vi "Set Finger Forces.vi"(8 "error in (no error)":errorcluster, 10 "Finger Forces":T1, 11 "MF3 in":refnum<class "MF3.lvclass">) -> (0 "error out":errorcluster, 2 "Current setpoints":dbl[](array[numeric]) format="%.2f", 3 "MF3 out":refnum<class "MF3.lvclass">)   [LabVIEW 2011, in "MF3.lvclass"]
uses:
  MF3.lvclass
  Controls/Motor Names.ctl
  MF3.lvclass/MF3.ctl
  <vilib>/Analysis/Matrix/Numeric/Multiply/Multiply - RM,RM.vi
  Finger/Finger.lvclass
  <vilib>/Analysis/Matrix/NI_Matrix.lvlib
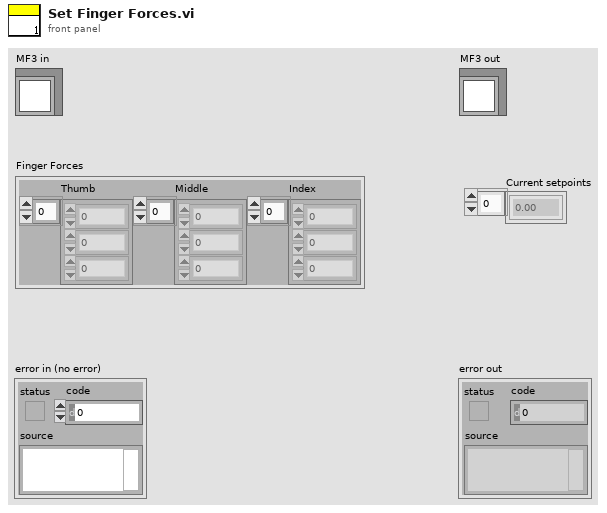
[diagram p1: front panel]
types:
  T1 = cluster{"Thumb":dbl[], "Middle":dbl[], "Index":dbl[]}
  T2 = typedef "Motor Names.ctl" = enum16{"Thumb1", "Thumb2", "Thumb3", "Middle1", "Middle2", "Middle3", "Redundant", "Index1", "Index2", "Index3"}
  T3 = typedef "NI_Matrix.lvlib/RealMatrix.ctl" = dbl[][]
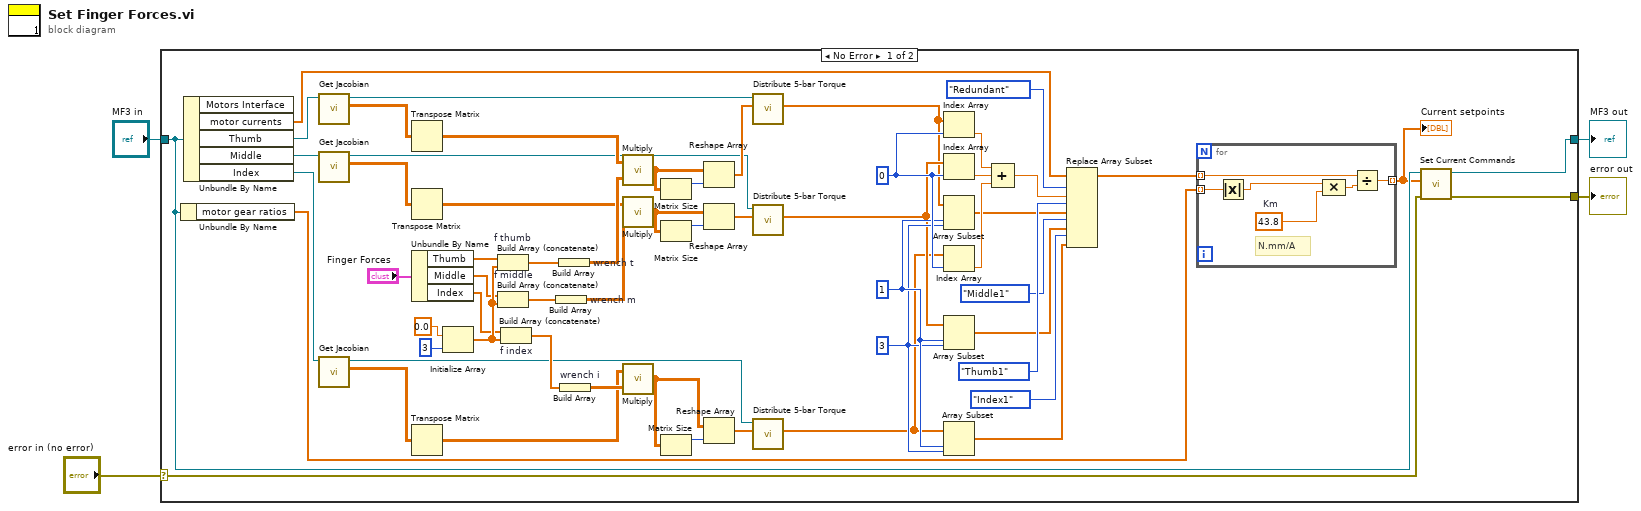
[diagram p0: block diagram]
diagram:
  n1 = case shown="No Error" "error in (no error)" {
    selector: "error in (no error)" -> [w8 w71]
    tunnel: [w7 w71] -> w3
    tunnel: [w6 w70] -> w1
    tunnel: "MF3 in" -> [w9 w70]
    frame No Error {
      w26 = 3 ("length")
      w27 = 1 ("index")
      w31 = 0 ("index")
      n2 = Unbundle By Name(w9) -> ("motor gear ratios"=w14:dbl[])
      n3 = Unbundle By Name(w9) -> ("motor currents"=w19:dbl[], "Thumb"=w63:refnum<class "Finger.lvclass">, "Middle"=w62:refnum<class "Finger.lvclass">, "Index"=w61:refnum<class "Finger.lvclass">)  [unwired: 1 out]
      n4 = call "Get Jacobian.vi"("Finger in"=w63) -> ("Jacobian"=w51:T3, "Finger out"=w35:refnum<class "Finger.lvclass">)  [unwired: 8 in, 1 out]
      n5 = call "Get Jacobian.vi"("Finger in"=w62) -> ("Jacobian"=w52:T3, "Finger out"=w34:refnum<class "Finger.lvclass">)  [unwired: 8 in, 1 out]
      n6 = call "Get Jacobian.vi"("Finger in"=w61) -> ("Jacobian"=w53:T3, "Finger out"=w33:refnum<class "Finger.lvclass">)  [unwired: 8 in, 1 out]
      n7 = Transpose Matrix(1:w51) -> (0:w50:T3)
      n8 = Transpose Matrix(1:w52) -> (0:w48:T3)
      n9 = Unbundle By Name("Finger Forces") -> ("Thumb"=w10:dbl[], "Middle"=w11:dbl[], "Index"=w12:dbl[])
      n10 = Transpose Matrix(1:w53) -> (0:w45:T3)
      n11 = Initialize Array(0.0 ("element"), 3 ("dimension size")) -> (w57:dbl[])
      n12 = Build Array (concatenate) "f thumb"(w10, w57) -> (w56:dbl[])
      n13 = Build Array (concatenate) "f middle"(w11, w57) -> (w55:dbl[])
      n14 = Build Array (concatenate) "f index"(w12, w57) -> (w54:dbl[])
      n15 = Build Array "wrench m"(w55) -> (w47:T3)
      n16 = Build Array "wrench t"(w56) -> (w49:T3)
      n17 = Build Array "wrench i"(w54) -> (w46:T3)
      n18 = call-poly <vilib>:"Multiply.vi"("Real Matrix B"=w49, "Real Matrix A"=w50) -> ("A * B"=w43:T3)
      n19 = call-poly <vilib>:"Multiply.vi"("Real Matrix B"=w47, "Real Matrix A"=w48) -> ("A * B"=w41:T3)
      n20 = call-poly <vilib>:"Multiply.vi"("Real Matrix B"=w46, "Real Matrix A"=w45) -> ("A * B"=w39:T3)
      n21 = Matrix Size(0:w43) -> (1:w44:i32)  [unwired: 1 out]
      n22 = Matrix Size(0:w41) -> (1:w42:i32)  [unwired: 1 out]
      n23 = Matrix Size(0:w39) -> (1:w40:i32)  [unwired: 1 out]
      n24 = Reshape Array(w43, w44) -> (w36:dbl[])
      n25 = Reshape Array(w41, w42) -> (w37:dbl[])
      n26 = Reshape Array(w39, w40) -> (w38:dbl[])
      n27 = call "Distribute 5-bar Torque.vi"("joint_torques"=w36, "Finger in"=w35) -> ("motor_torques"=w23:dbl[])  [unwired: 7 in, 2 out]
      n28 = call "Distribute 5-bar Torque.vi"("joint_torques"=w37, "Finger in"=w34) -> ("motor_torques"=w25:dbl[])  [unwired: 7 in, 2 out]
      n29 = call "Distribute 5-bar Torque.vi"("joint_torques"=w38, "Finger in"=w33) -> ("motor_torques"=w24:dbl[])  [unwired: 7 in, 2 out]
      n30 = Index Array(array=w23, index=w31) -> (element=w32:dbl)
      n31 = Index Array(array=w25, index=w31) -> (element=w29:dbl)
      n32 = Array Subset(array=w23, index=w27, length=w26) -> (w17:dbl[])
      n33 = Index Array(array=w24, index=w31) -> (element=w30:dbl)
      n34 = Array Subset(array=w25, index=w27, length=w26) -> (w16:dbl[])
      n35 = Array Subset(array=w24, index=w27, length=w26) -> (w15:dbl[])
      n36 = Compound Arithmetic op=ADD(w32, w29, w30) -> (w18:dbl)
      n37 = Replace Array Subset "Replace Array Subset"(array=w19, new element #1=w18, index #1=Motor_Names."Redundant" ("Motor Names"), new element #2=w17, index #2=Motor_Names."Thumb1" ("Motor Names"), new element #3=w16, index #3=Motor_Names."Middle1" ("Motor Names"), new element #4=w15, index #4=Motor_Names."Index1" ("Motor Names")) -> (w13:dbl[])
      n38 = for {
        tunnel: w14 -> [w65] mode=indexing
        tunnel: w13 -> [w69] mode=indexing
        tunnel: [w67] -> w5 mode=indexing
        w64 = 43.8  # Km
        # "N.mm/A"
        n39 = Absolute Value(x=w65) -> (abs(x)=w66:dbl)
        n40 = Compound Arithmetic op=MULTIPLY(w66, w64) -> (w68:dbl)
        n41 = Divide(x=w69, y=w68) -> (x/y=w67:dbl)
      }
      "Current setpoints" <- w5
      n42 = call "Set Current Commands.vi"("error in (no error)"=w8, "current commands"=w5, "MF3 in"=w9) -> ("error out"=w7:errorcluster, "MF3 out"=w6:refnum<class "MF3.lvclass">)  [unwired: 7 in]
    }
    frame Error {
    }
  }
  "error out" <- w3
  "MF3 out" <- w1
